vi "2.计数器Counters.vi"() -> ()   [LabVIEW 2019]
uses:
  <vilib>/rvi/Emulation/niFpgaGetClockAttributes.vi
  <vilib>/rvi/Emulation/niFpgaSctlEmulationGetInTimedLoop.vi
  <vilib>/rvi/Emulation/niFpgaEmulationReportErrorSimple.vi
  <vilib>/rvi/eio/common/nirviEmuTemplateMethod_errors.vi
  <vilib>/rvi/Emulation/niFpgaCriticalErrorInLSC.vi
  <vilib>/eio/EIONode/EIONode.xnode
panel:
  out "Counters":u8
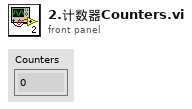
[diagram p1: front panel]
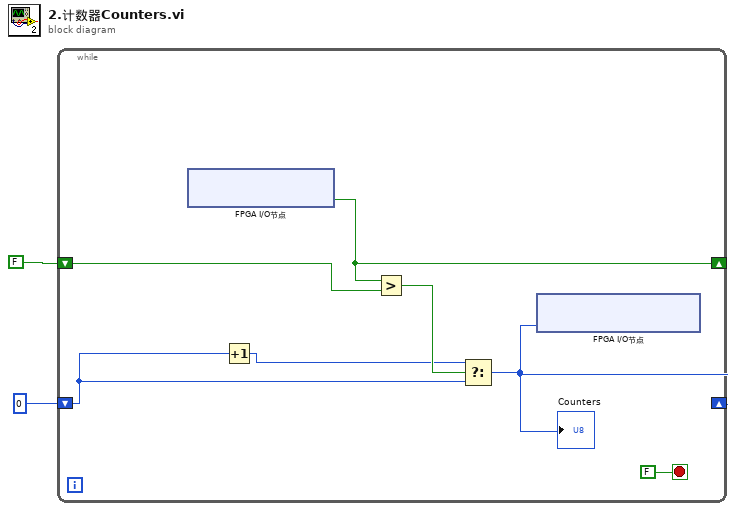
[diagram p0: block diagram]
diagram:
  n1 = while {
    shift-right: [w7] -> _
    shift-left: FALSE -> [w8]
    shift-right: [w3] -> _
    shift-left: u8 0 -> [w4]
    stop <- FALSE stop-if-true
    n2 = xnode "FPGA I/O节点"() -> ("ConnectorA/DIO1"=w7:bool)  [unwired: 1 in, 1 out]
    n3 = Increment(x=w4) -> (x+1=w5:u8)
    n4 = Greater?(x=w7, y=w8) -> (0:w6:bool)
    n5 = Select(t=w5, s=w6, f=w4) -> (s? t:f=w3:u8)
    "Counters" <- w3
    n6 = xnode "FPGA I/O节点"("ConnectorA/DIO15:8"=w3) -> ()  [unwired: 1 in, 1 out]
  }
